vi "Set PMTs.vi"(8 "Error In":errorcluster, 10 "PMT 2":T1 max=1000 step=5 scale=0.0..1000.0, 11 "PMT 1":T1 max=1000 step=5 scale=0.0..1000.0) -> (0 "Error Out":errorcluster)   [LabVIEW 2020]
uses:
  Typedefs/HW config states enum.ctl
  <vilib>/DAQmx/create/channels.llb/DAQmx Create Channel (AO-Voltage-Basic).vi
  <vilib>/DAQmx/write.llb/DAQmx Write (Analog 1D DBL NChan 1Samp).vi
  Typedefs/PMT control knob.ctl
panel:
  out "DAQmx Physical Channel":tag="PXI1Slot4/ao2:3"
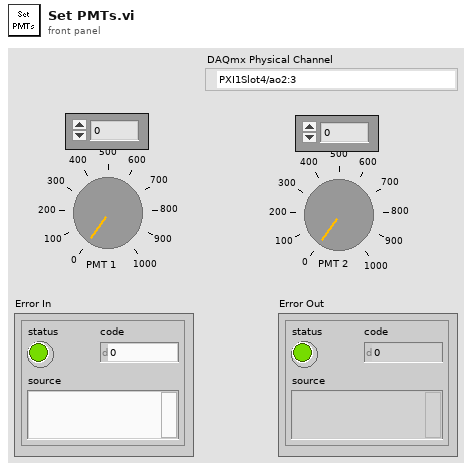
[diagram p1: front panel]
types:
  T1 = typedef "PMT control knob.ctl" = u16
  T2 = typedef "HW config states enum.ctl" = enum16{"Load from file", "Save to file", "Save backup", "Write all", "Read all", "Write XY stage settings", "Write DAQ FPGA settings", "Write Control FPGA settings", "Write Phys Channels", "Write System Config", "Write HW Config", "Save System Config", "Save HW Config", "Clear", "Compare from file"}
  T3 = typedef "Hardware Configuration settings.ctl" = cluster{"Dev. PC":bool, "Swap XY on stage":bool, "No of AOD":u8, "MC Supported":bool, "Axial MC":bool, "Computer MAC address":string, "Externalise Triggers":bool, "Trigger HW config":T4, "DAQmx Chan":T5, "XYZ Stage Control Config":T6, "XY stage available":bool, "XY Comms Config Cluster":T7, "Y stage available":bool, "Y Comms Config Cluster":T7, "Z stage available":bool, "Z Comms Config Cluster ":T7, "Encoder available":bool, "Encoder":T9, "VidRec available":bool, "Cam VidRec":T10, "Laser Power Control HW config":T11, "Laser 1 available":bool, "Laser 1 config cluster":T12, "Prechirper 1 available":bool, "Prechirper 1 config cluster":T13, "Control system.FPGA available?":bool, "Control Sys. HW config":T14, "DAQ FPGA HW Config":T15, "PMT Control Voltage Limits":T19}
  T4 = typedef "Triggers HW config.ctl" = cluster{"Available Device List":i32, "Device Address":string}
  T5 = typedef "DAQmx physical channels cluster.ctl" = cluster{"Pockels AO":tag, "Hard shutter AO":tag, "PMT AOs":tag, "Galvo AOs":tag, "Power meter AI":tag}
  T6 = typedef "XYZControlConfig.ctl" = enum16{"None", "XYZ", "XY-Z", "X-Y-Z", "Z"}
  T7 = typedef "Peripherals comms config cluster.ctl" = cluster{"Name":string, "Device Address":string, "Port ":u16, "Baudrate":i32, "Comms Type":T8}
  T8 = typedef "Comms Type.ctl" = enum16{"GPIB-IEEE488", "Serial-RS232", "Serial-RS485", "Serial-RS422", "Serial-USB", "Ethernet-TCP/IP", "Ethernet-UDP"}
  T9 = typedef "Encoder config cluster.ctl" = cluster{"IP address":string, "Port":u16, "Wheel radius (cm)":dbl, "Encoder Trigger":tag}
  T10 = typedef "Cam VidRec HW config setup cluster.ctl" = cluster{"DO flag-Video record":tag, "DO flag-Trial start":tag}
  T11 = typedef "Laser Power Control HW config.ctl" = cluster{"Laser Power Control":string, "Laser Power Modulation Control":enum16{"NI", "FPGA"}}
  T12 = typedef "Laser 1 config cluster.ctl" = cluster{"COM port":refnum<visa-resource-name>, "Baud Rate":i32, "Type":string}
  T13 = typedef "PreChirper 1 config cluster.ctl" = cluster{"Type":string, "Baud Rate":i32, "COM port":refnum<visa-resource-name>}
  T14 = typedef "Control Sys HW config cluster.ctl" = cluster{"Control system.FPGA Type":enum16{"Virtex 5", "Virtex 7"}, "Control system.Network adapter name":string, "Control system.MAC address":string, "Control system.Ethernet Port":u32, "Control system.Ethernet Port Opened":bool}
  T15 = typedef "DAQ FPGA HW config cluster.ctl" = cluster{"FGPA Ref":T16, "Target":T17, "input card type":T18}
  T16 = typedef "FPGA Ref.ctl" = refnum<k20>
  T17 = typedef "nirio_resource_hc.ctl" = tag
  T18 = typedef "FPGA input type AC-DC.ctl" = enum16{"AC Card", "DC Card"}
  T19 = typedef "PMT Control Voltage limits.ctl" = cluster{"Lower Limit":dbl, "Upper Limit":dbl}
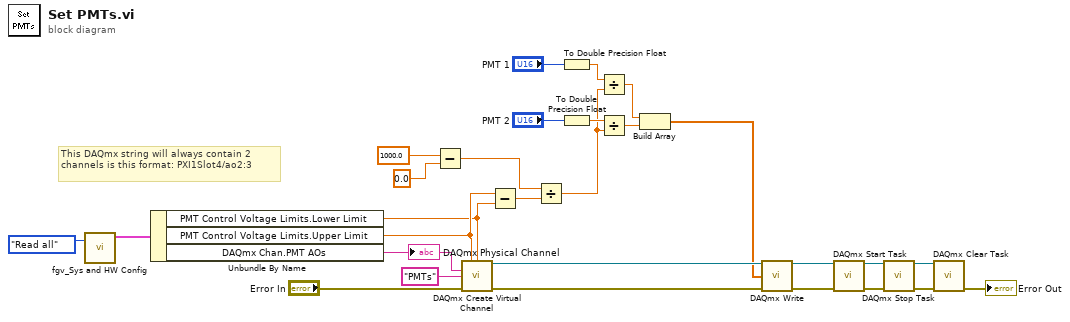
[diagram p0: block diagram]
diagram:
  # "This DAQmx string will always contain 2 channels is this format: PXI1Slot4/ao2:3"
  n1 = call "fgv_Sys and HW Config.vi"("Function"=HW_config_states_enum."Read all") -> ("Hardware Configuration OUT"=w9:T3)  [unwired: 8 in, 2 out]
  n2 = Unbundle By Name(w9) -> ("PMT Control Voltage Limits.Lower Limit"=w6:dbl, "PMT Control Voltage Limits.Upper Limit"=w7:dbl, "DAQmx Chan.PMT AOs"=w8:tag)
  "DAQmx Physical Channel" <- w8
  n3 = Subtract(x=1000.0, y=0.0) -> (x-y=w1:dbl)
  n4 = call-poly <vilib>:"DAQmx Create Virtual Channel.vi"("maximum value"=w7, "minimum value"=w6, "physical channels"=w8, "name to assign"="PMTs", "error in"="Error In") -> ("task out"=w28:refnum<k21>, "error out"=w27:errorcluster)  [unwired: 9 in]
  n5 = Subtract(x=w7, y=w6) -> (x-y=w2:dbl)
  n6 = Divide(x=w1, y=w2) -> (x/y=w5:dbl)
  n7 = To Double Precision Float(number="PMT 1") -> (double precision float=w11:dbl)
  n8 = To Double Precision Float(number="PMT 2") -> (double precision float=w12:dbl)
  n9 = Divide(x=w11, y=w5) -> (x/y=w17:dbl)
  n10 = Divide(x=w12, y=w5) -> (x/y=w14:dbl)
  n11 = Build Array(w17, w14) -> (w13:dbl[])
  n12 = call-poly <vilib>:"DAQmx Write.vi"("task/channels in"=w28, "data"=w13, "error in"=w27) -> ("task out"=w26:refnum<k21>, "error out"=w25:errorcluster)  [unwired: 10 in, 1 out]
  n13 = call <vilib>:"DAQmx Start Task.vi"("task/channels in"=w26, "error in"=w25) -> ("task out"=w19:refnum<k21>, "error out"=w20:errorcluster)  [unwired: 12 in]
  n14 = call <vilib>:"DAQmx Stop Task.vi"("task/channels in"=w19, "error in"=w20) -> ("task out"=w24:refnum<k21>, "error out"=w23:errorcluster)  [unwired: 12 in]
  n15 = call <vilib>:"DAQmx Clear Task.vi"("task in"=w24, "error in"=w23) -> ("error out"=→"Error Out":errorcluster)  [unwired: 13 in]
